vi "Configure Calibration Kit.vi"(0 "VISA resource name":refnum<visa-resource-name>, 1 "C0 (0.0)":dbl format="%^.2e", 3 "C1  (0.0)":dbl format="%^.2e", 4 "C2  (0.0)":dbl format="%^.2e", 5 "C3  (0.0)":dbl format="%^.2e", 7 "error in (no error)":errorcluster, 8 "Channel (1)":i32=1, 9 "L0  (0.0)":dbl format="%^.2e", 11 "L1  (0.0)":dbl format="%^.2e", 12 "Standard (1)":i32=1, 13 "L2  (0.0)":dbl format="%^.2e", 14 "Label (\"Name\")":string="Name", 15 "L3  (0.0)":dbl format="%^.2e", 16 "Type (0: Open)":u16(ring) items=["Open", "Short", "Load", "Thru", "Arbitrary Impedance", "DUT of which theoretical values are 0", "Unknown Thru"], 18 "Arbitrary Impedance  (0.0)":dbl format="%^.2e", 19 "Cal Kit Name (\"Cal1\")":string="Cal1") -> (20 "VISA resource name out":refnum<visa-resource-name>, 27 "error out":errorcluster)   [LabVIEW 2011, in "Agilent ENA Series.lvlib"]
doc: "This VI configures calibration kit standard."
uses:
  Agilent ENA Series.lvlib
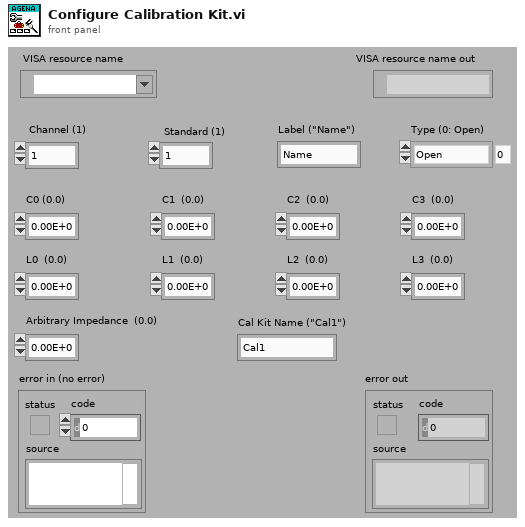
[diagram p1: front panel]
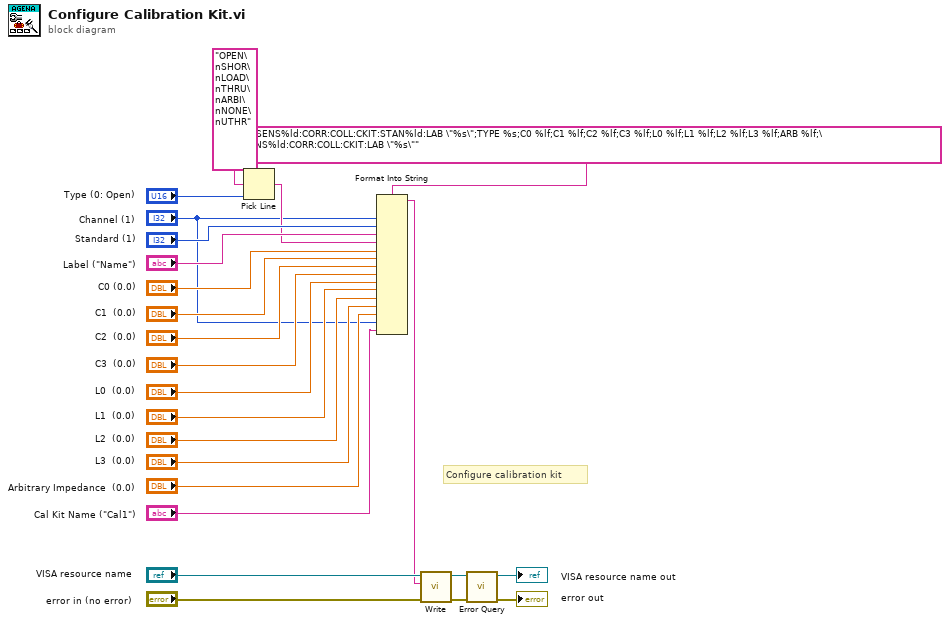
[diagram p0: block diagram]
diagram:
  # "Configure calibration kit"
  n1 = Pick Line(multi-line string="OPEN\nSHOR\nLOAD\nTHRU\nARBI\nNONE\nUTHR", line index="Type (0: Open)") -> (output string=w16:string)  [unwired: 1 in]
  n2 = Format Into String(format string="%.;:SENS%ld:CORR:COLL:CKIT:STAN%ld:LAB \"%s\";TYPE %s;C0 %lf;C1 %lf;C2 %lf;C3 %lf;L0 %lf;L1 %lf;L2 %lf;L3 %lf;ARB %lf;\n:SENS%ld:CORR:COLL:CKIT:LAB \"%s\"", "Channel (1)", "Standard (1)", "Label (\"Name\")", w16, "C0 (0.0)", "C1  (0.0)", "C2  (0.0)", "C3  (0.0)", "L0  (0.0)", "L1  (0.0)", "L2  (0.0)", "L3  (0.0)", "Arbitrary Impedance  (0.0)", "Channel (1)", "Cal Kit Name (\"Cal1\")") -> (resulting string=w21:string)  [unwired: 2 in, 1 out]
  n3 = call "Write.vi"("error in (no error)"="error in (no error)", "String ()"=w21, "VISA resource name"="VISA resource name") -> ("error out"=w5:errorcluster, "VISA resource name out"=w6:refnum<visa-resource-name>)  [unwired: 6 in, 1 out]
  n4 = call "Error Query.vi"("error in (no error)"=w5, "VISA resource name"=w6) -> ("error out"=→"error out":errorcluster, "VISA resource name out"=→"VISA resource name out":refnum<visa-resource-name>)  [unwired: 6 in, 2 out]
